vi "MultipleActionEngineSANDBOX.vi"() -> ()   [LabVIEW 2022 SP3]
uses:
  ActionEngineEnum.ctl
  C:/Users/ulate/Documents/mnOP/mnOPSuite-main/PRISM/Thorlabs.MotionControl.Controls.dll
  mnOPSuite-main/PRISM/Thorlabs.MotionControl.Controls.dll
panel:
  in  "Stop All":bool
  in  "KCubeStepperControl 2":refnum<k24>(container)
  in  "SerialNumber 2":string="26004239"
  in  "Position Settings 2":T1={"Step Size (mm)"=10.0, "Initial Position"=0.0, "Num Of Steps"=200, "Move Position"=0.0, "Step Delay (ms)"=0} {"Step Size (mm)" min=0.00046 format="%.8f"}
  out "Current Position 2":dbl
  out "error out 2":errorcluster
  in  "Action 2":T2=enum."Done"
  in  "stop 2":bool
  in  "Use \"DONE\" as Stop 2":bool=TRUE
  in  "stop":bool
  in  "Use \"DONE\" as Stop":bool=TRUE
  in  "Action":T2=enum."Done"
  out "error out":errorcluster
  out "Current Position":dbl
  in  "Position Settings":T1={"Step Size (mm)"=10.0, "Initial Position"=0.0, "Num Of Steps"=200, "Move Position"=0.0, "Step Delay (ms)"=0} {"Step Size (mm)" min=0.00046 format="%.8f"}
  in  "SerialNumber":string="26004239"
  in  "KCubeStepperControl":refnum<k24>(container)
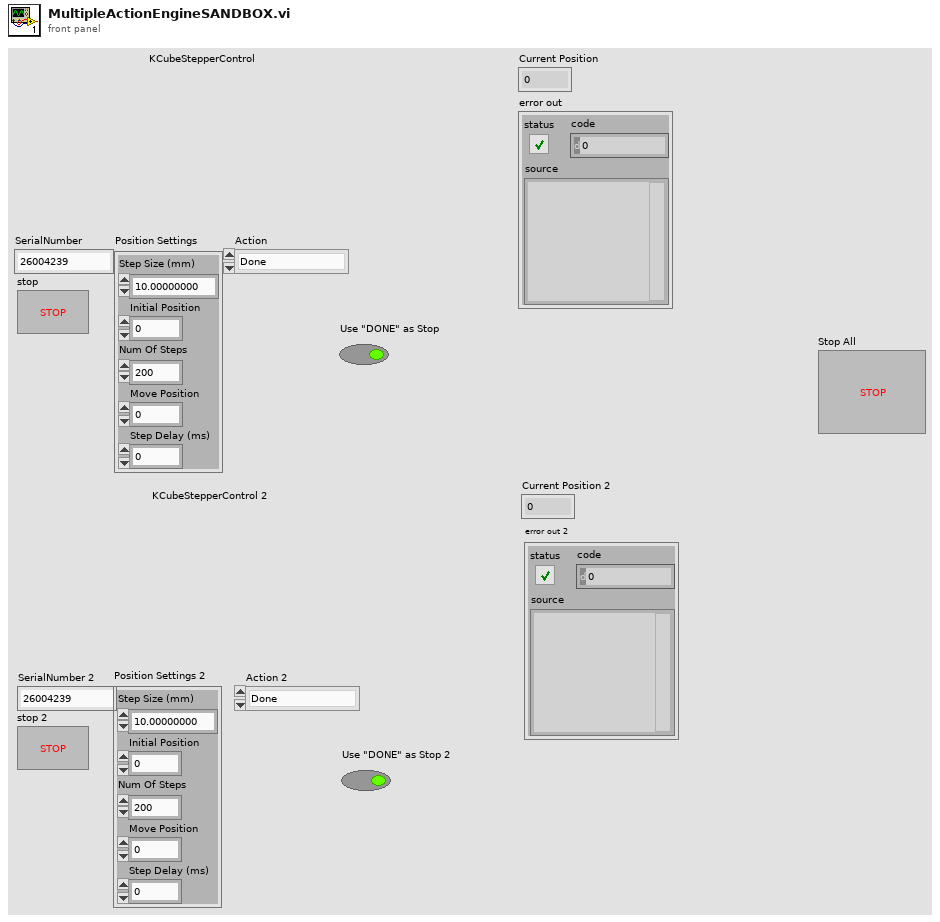
[diagram p1: front panel]
types:
  T1 = cluster{"Step Size (mm)":sgl, "Initial Position":dbl, "Num Of Steps":i32, "Move Position":dbl, "Step Delay (ms)":u32}
  T2 = typedef "ActionEngineEnum.ctl" = enum16{"Open Connection", "Done", "Get Position", "Settings", "Home", "Move Absolute", "Move Relative", "Step", "Close Connection"}
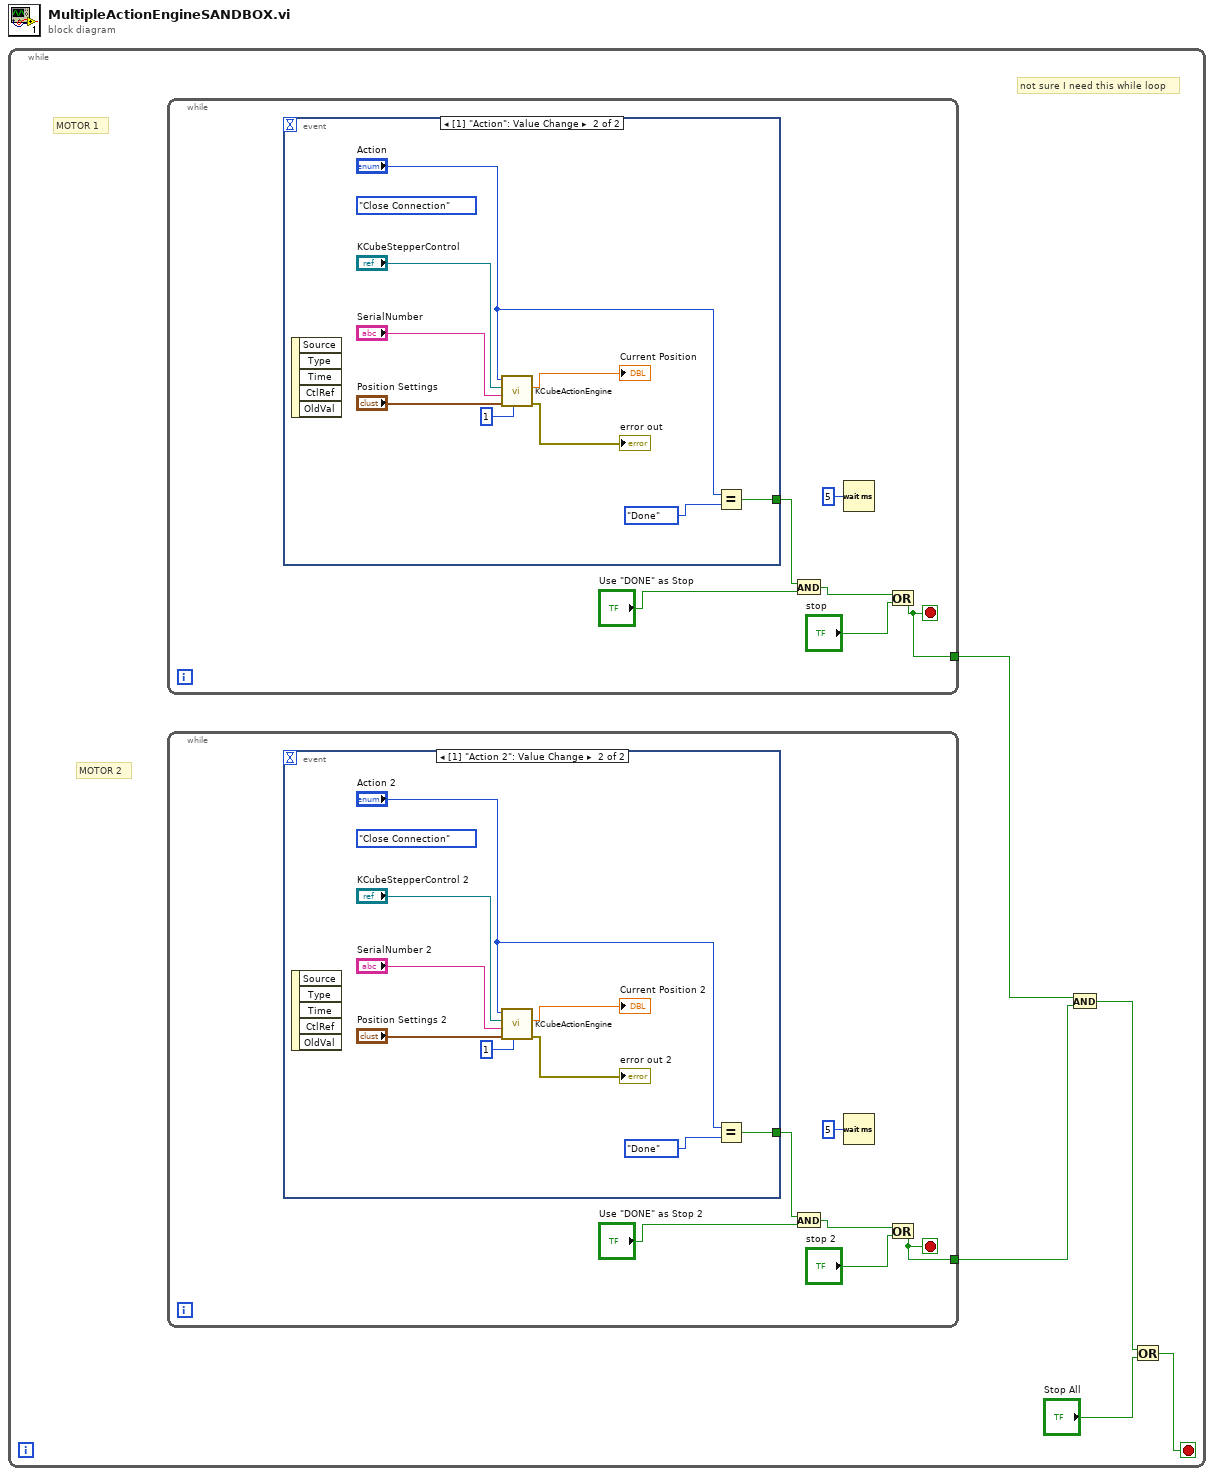
[diagram p0: block diagram]
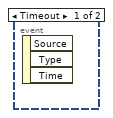
[diagram p2: hidden frame]
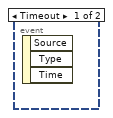
[diagram p3: hidden frame]
diagram:
  n1 = while {
    stop <- w1 stop-if-true
    # "not sure I need this while loop"
    # "MOTOR 2"
    # "MOTOR 1"
    n2 = while {
      tunnel: [w21] -> w5
      stop <- w21 stop-if-true
      n3 = event shown="[1] \"Action\": Value Change" {
        selector: _ -> [_ _]
        dyn-events: _ -> [_ _]
        timeout: _ -> [_ _]
        tunnel: [_ w27] -> w22
        event Timeout {
          n4 = event-data() -> ()  [unwired: 1 in, 3 out]
        }
        event Value Change {
          (unwired) ActionEngineEnum."Close Connection" ("Action")
          n5 = event-data() -> ()  [unwired: 1 in, 5 out]
          n6 = call "KCubeActionEngine.vi"("ChannelNumber"=1, "Position Settings"="Position Settings", "SerialNumber"="SerialNumber", "KCubeStepperControl"="KCubeStepperControl", "Action"="Action") -> ("error out"=→"error out":errorcluster, "Current Position"=→"Current Position":dbl)  [unwired: 4 in]
          n7 = Equal?(x="Action", y=ActionEngineEnum."Done" ("Action")) -> (x = y?=w27:bool)
        }
      }
      n8 = And(x=w22, y="Use \"DONE\" as Stop") -> (x .and. y?=w26:bool)
      n9 = Wait (ms)(milliseconds to wait=u32 5) -> ()  [unwired: 1 out]
      n10 = Or(x=w26, y="stop") -> (x .or. y?=w21:bool)
    }
    n11 = while {
      tunnel: [w6] -> w4
      stop <- w6 stop-if-true
      n12 = event shown="[1] \"Action 2\": Value Change" {
        selector: _ -> [_ _]
        dyn-events: _ -> [_ _]
        timeout: _ -> [_ _]
        tunnel: [_ w12] -> w7
        event Timeout {
          n13 = event-data() -> ()  [unwired: 1 in, 3 out]
        }
        event Value Change {
          (unwired) ActionEngineEnum."Close Connection" ("Action")
          n14 = event-data() -> ()  [unwired: 1 in, 5 out]
          n15 = call "KCubeActionEngine.vi"("ChannelNumber"=1, "Position Settings"="Position Settings 2", "SerialNumber"="SerialNumber 2", "KCubeStepperControl"="KCubeStepperControl 2", "Action"="Action 2") -> ("error out"=→"error out 2":errorcluster, "Current Position"=→"Current Position 2":dbl)  [unwired: 4 in]
          n16 = Equal?(x="Action 2", y=ActionEngineEnum."Done" ("Action")) -> (x = y?=w12:bool)
        }
      }
      n17 = And(x=w7, y="Use \"DONE\" as Stop 2") -> (x .and. y?=w11:bool)
      n18 = Wait (ms)(milliseconds to wait=u32 5) -> ()  [unwired: 1 out]
      n19 = Or(x=w11, y="stop 2") -> (x .or. y?=w6:bool)
    }
    n20 = And(x=w5, y=w4) -> (x .and. y?=w2:bool)
    n21 = Or(x=w2, y="Stop All") -> (x .or. y?=w1:bool)
  }
